vi "FTW-ERR-Assert-Truthy.vi"(7 "Expected Truthy":bool, 11 "error in":errorcluster) -> (15 "error out":errorcluster)   [LabVIEW 2014]
uses:
  FTW-ERR-ThrowError.vi
  FTW-ERR-NoErrorConstant.vi
  string/FTW-STR-ReplaceWhitespace.vi
  FTW-ERR-CallChain.vi
panel:
  # "Inputs"
  # "Outputs"
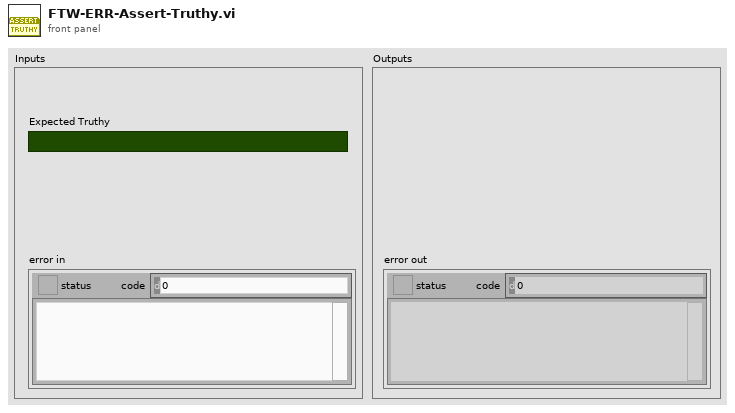
[diagram p1: front panel]
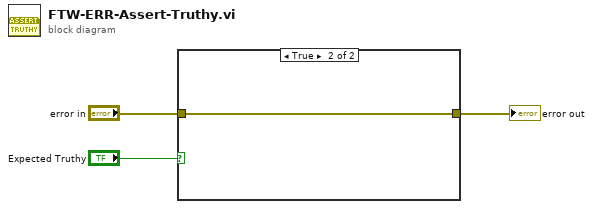
[diagram p0: block diagram]
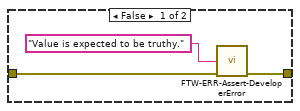
[diagram p2: hidden frame]
diagram:
  n1 = case shown="True" "Expected Truthy" {
    tunnel: "error in" -> [w5 w7]
    tunnel: [w4 w7] -> w2
    frame False {
      n2 = call "FTW-ERR-Assert-DeveloperError.vi"("Reason this error should never happen"="Value is expected to be truthy.", "error in"=w5) -> ("error out"=w4:errorcluster)  [unwired: 13 in]
    }
    frame True {
    }
  }
  "error out" <- w2
